vi "Calculate Force Calibration Linear Fit.vi"(8 "error in (no error)":errorcluster, 11 "array results in":T1) -> (0 "error out":errorcluster, 2 "new results?":bool, 3 "array results out":T1)   [LabVIEW 2020]
uses:
  Controller Loop/Controller Data.ctl
  <vilib>/Analysis/NI_AALPro.lvlib
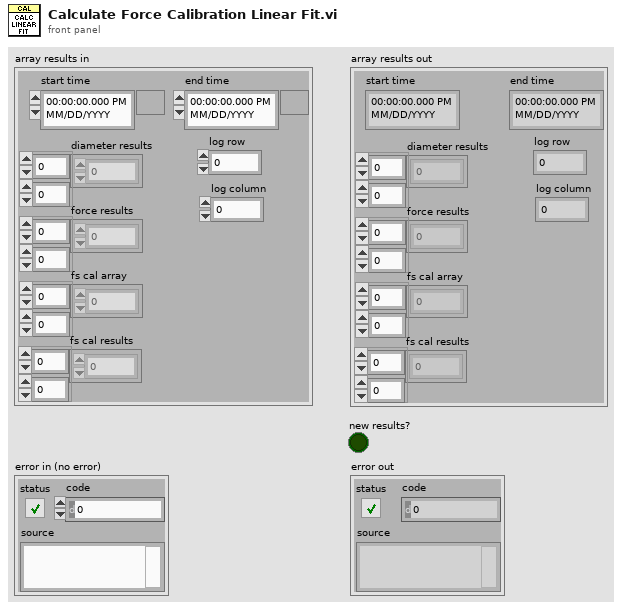
[diagram p1: front panel]
types:
  T1 = typedef "Controller Data.ctl" = cluster{"diameter results":dbl[][], "force results":dbl[][], "fs cal array":dbl[][], "fs cal results":dbl[][], "start time":timestamp, "end time":timestamp, "log row":i32, "log column":i32}
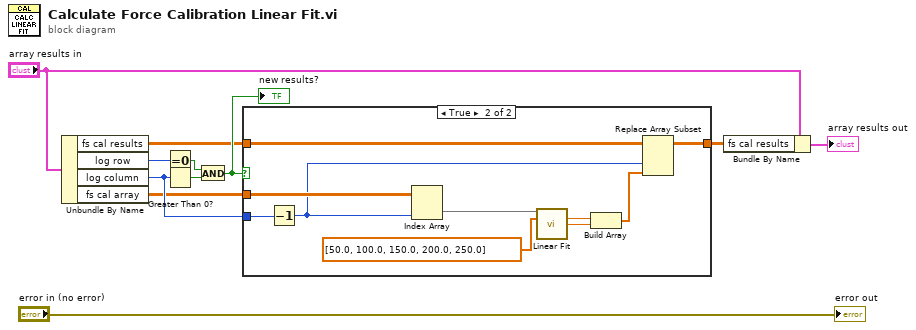
[diagram p0: block diagram]
diagram:
  n1 = Unbundle By Name("array results in") -> ("fs cal results"=w2:dbl[][], "log row"=w9:i32, "log column"=w5:i32, "fs cal array"=w4:dbl[][])
  n2 = Equal To 0?(x=w9) -> (x = 0?=w8:bool)
  n3 = Greater Than 0?(x=w5) -> (x > 0?=w7:bool)
  n4 = And(x=w8, y=w7) -> (x .and. y?=w6:bool)
  "new results?" <- w6
  n5 = case shown="True" w6 {
    tunnel: w5 -> [_ w22]
    tunnel: w4 -> [_ w21]
    tunnel: w2 -> [w12 w20]
    tunnel: [w12 w19] -> w1
    frame False {
    }
    frame True {
      n6 = Decrement(x=w22) -> (x-1=w18:i32)
      n7 = Index Array(array=w21, index (col)=w18) -> (element=w13:dbl[])  [unwired: 1 in]
      n8 = call <vilib>:"Linear Fit.vi"("Y"=w13, "X"=dbl[] [50.0, 100.0, 150.0, 200.0, 250.0] ("Y")) -> ("slope"=w17:dbl, "intercept"=w16:dbl)  [unwired: 9 in, 3 out]
      n9 = Build Array(w17, w16) -> (w15:dbl[])
      n10 = Replace Array Subset(array=w20, new element=w15, index (col)=w18) -> (w19:dbl[][])  [unwired: 1 in]
    }
  }
  n11 = Bundle By Name(cluster="array results in", "fs cal results"=w1) -> (→"array results out":T1)
  "error out" <- "error in (no error)"
